vi "CC Rd Wr Hardware Configuration.vi"(8 "error in (no error)":errorcluster, 10 "Write? (F:Read)":bool, 11 "Hardware Config":T1) -> (0 "error out":errorcluster, 1 "New File?":bool, 2 "File":path, 3 "Hardware Config out":T1)   [LabVIEW 2024]
uses:
  typedefs/CC cluster Hardware Config.ctl
  typedefs/CC cluster Device Index.ctl
  2e80df6d-94aa-46b9-8b94-ceea8c057880.vi
  659fb017-0e9f-42f9-b06e-930303f00cbc.vi
  <vilib>/JDP Science/JSONtext/Find Item.vi
  <vilib>/JDP Science/JSONtext/Next JSON Value.vi
  <vilib>/JDP Science/JSONtext/String Subset.vi
  <vilib>/JDP Science/JSONtext/Parsing/Advance past next JSON Value (inlined COPY).vi
  <vilib>/JDP Science/JSONtext/Parsing/Advance past whitespace.vi
  <vilib>/JDP Science/JSONtext/Parsing/Advance past String.vi
  <vilib>/JDP Science/JSONtext/Parsing/Advance past Number.vi
  <vilib>/JDP Science/JSONtext/Parsing/Advance past Line Ending.vi
  <vilib>/JDP Science/JSONtext/Parsing/Parse Full Path or Item Name.vi
  <vilib>/JDP Science/JSONtext/Parsing/Advance past Array.vi
  <vilib>/JDP Science/JSONtext/Parsing/Advance past Object.vi
  <vilib>/JDP Science/JSONtext/support/Error Cluster From Code.vi
  <vilib>/JDP Science/JSONtext/Offset/Find Item Locations by Path.vi
  <vilib>/JDP Science/JSONtext/JSON text to Variant.vi
  <vilib>/JDP Science/JSONtext/Variant to JSON Text.vi
  <vilib>/JDP Science/JSONtext/Set Item.vi
  <vilib>/JDP Science/JSONtext/LVClass Serializer/JSONtext LVClass Serializer.lvclass
panel:
  in  "Settings File":string="CC System Settings.json"
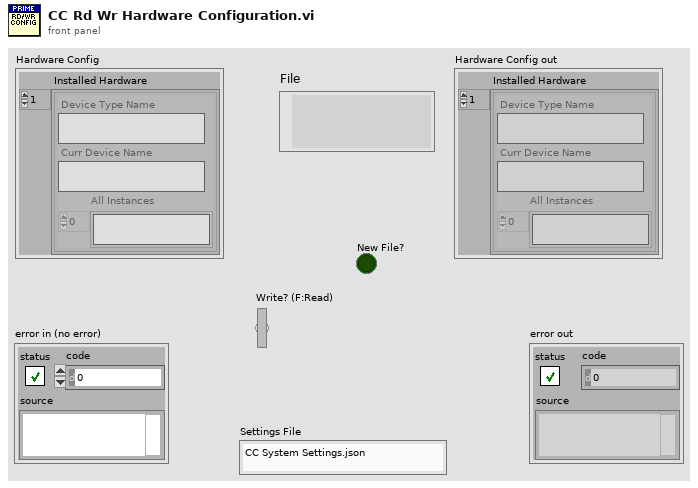
[diagram p1: front panel]
types:
  T1 = typedef "CC cluster Hardware Config.ctl" = cluster{"Installed Hardware":T2[]}
  T2 = typedef "CC cluster Device Index.ctl" = cluster{"Device Type Name":string, "Curr Device Name":string, "All Instances":string[]}
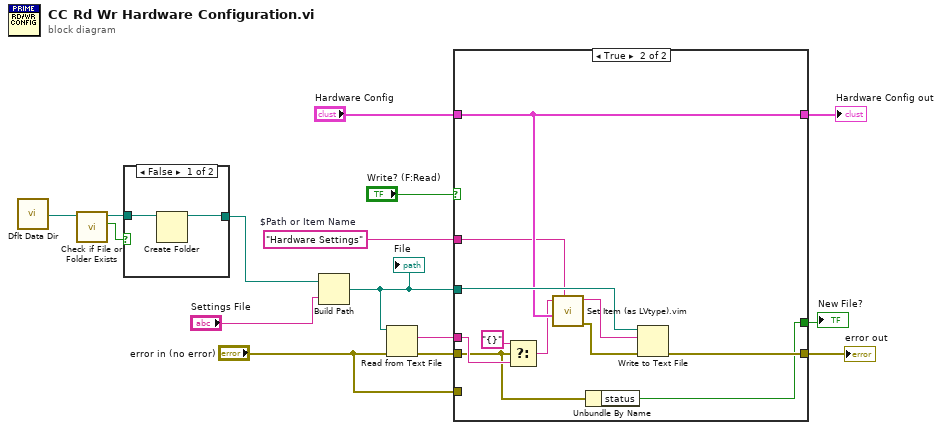
[diagram p0: block diagram]
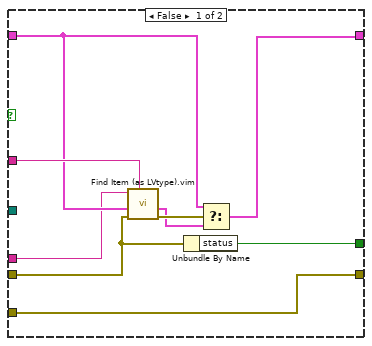
[diagram p3: hidden frame]
diagram:
  w10 = "Hardware Settings"  # $Path or Item Name
  n1 = call <vilib>:"Dflt Data Dir.vi"() -> ("App:Default Data Directory"=w4:path)
  n2 = call <vilib>:"Check if File or Folder Exists.vi"("path"=w4) -> ("file or folder exists?"=w3:bool, "dup path"=w2:path)  [unwired: 8 in, 1 out]
  n3 = case shown="False" w3 {
    tunnel: w2 -> [w17 w18]
    tunnel: [w16 w18] -> w1
    frame False {
      n4 = Create Folder(path (use dialog)=w17) -> (created path=w16:path)  [unwired: 2 in, 2 out]
    }
    frame True {
    }
  }
  n5 = Build Path(base path=w1, name or relative path="Settings File") -> (appended path=w7:path)
  "File" <- w7
  n6 = Read from Text File(file (use dialog)=w7, error in="error in (no error)") -> (text=w8:string, error out=w9:errorcluster)  [unwired: 2 in, 2 out]
  n7 = case shown="True" "Write? (F:Read)" {
    tunnel: w9 -> [w20 w29]
    tunnel: "Hardware Config" -> [w25 w36]
    tunnel: w7 -> [_ w38]
    tunnel: [w21 w37] -> w13
    tunnel: [w27 w36] -> w12
    tunnel: w10 -> [w26 w35]
    tunnel: w8 -> [w22 w32]
    tunnel: "error in (no error)" -> [w21 _]
    tunnel: [w19 w28] -> w5
    frame False {
      n8 = call "Find Item (as LVtype).vim"("$Path or Item Name"=w26, "error in (no error)"=w20, "Data Type and Default Value"=w25, "JSON"=w22) -> ("error out"=w24:errorcluster, "Data"=w23:T1)  [unwired: 4 in, 2 out]
      n9 = Unbundle By Name(w20) -> ("status"=w19:bool)
      n10 = Select(t=w25, s=w24, f=w23) -> (s? t:f=w27:T1)
    }
    frame True {
      n11 = Select(t="{}" ("JSON"), s=w29, f=w32) -> (s? t:f=w31:string)
      n12 = call "Set Item (as LVtype).vim"("$Path or Item Name"=w35, "Anything"=w36, "JSON"=w31) -> ("error out"=w30:errorcluster, "<JSON>"=w34:string)  [unwired: 5 in, 1 out]
      n13 = Unbundle By Name(w29) -> ("status"=w28:bool)
      n14 = Write to Text File(file (use dialog)=w38, text=w34, error in=w30) -> (error out=w37:errorcluster)  [unwired: 1 in, 2 out]
    }
  }
  "error out" <- w13
  "Hardware Config out" <- w12
  "New File?" <- w5
